vi "Table_ResizeListbox.vi"(7 "VI in":refnum<vi>, 8 "error in (no error)":errorcluster, 10 "Listbox Ref":refnum<vi>, 11 "State Information":T1) -> (0 "error out":errorcluster, 2 "Listbox Ref Out":refnum<vi>, 3 "State Information Out":T1)   [LabVIEW 2012, in "TableSupportLib.lvlib"]
uses:
  TableSupportLib.lvlib
  Table_StateInformation.ctl
  Table_ChannelInfoCluster.ctl
  Table_SortArraySettings.ctl
  Table_ListboxSettings.ctl
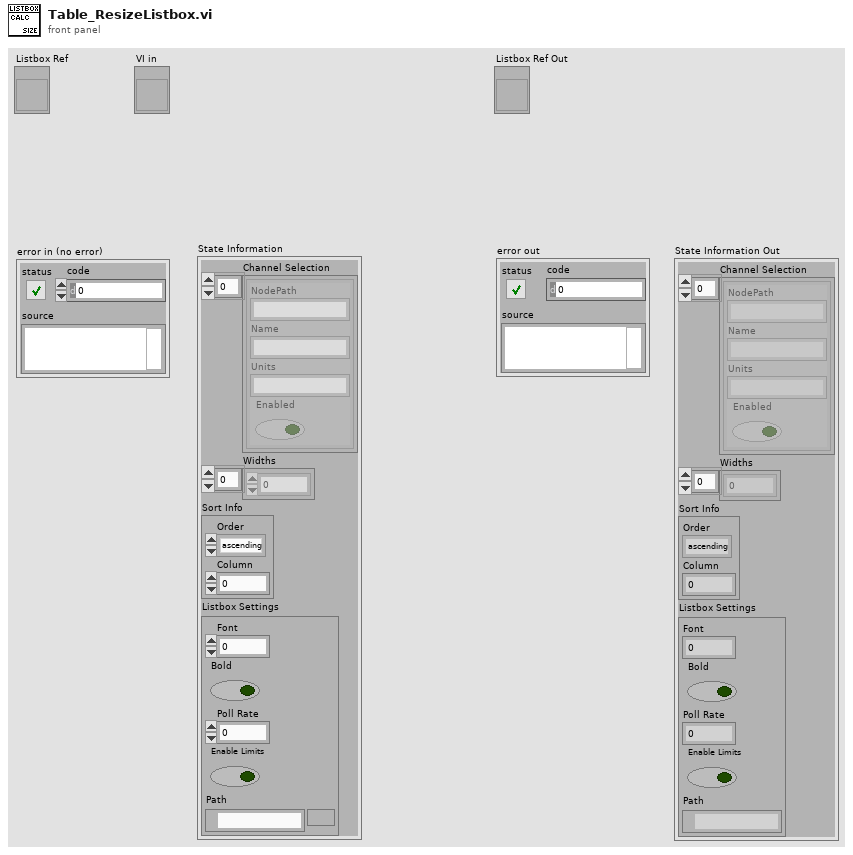
[diagram p1: front panel]
types:
  T1 = typedef "TableSupportLib.lvlib/Table_StateInformation.ctl" = cluster{"Channel Selection":T2[], "Widths":dbl[], "Sort Info":T3, "Listbox Settings":T4}
  T2 = typedef "TableSupportLib.lvlib/Table_ChannelInfoCluster.ctl" = cluster{"NodePath":string, "Name":string, "Units":string, "Enabled":bool}
  T3 = typedef "TableSupportLib.lvlib/Table_SortArraySettings.ctl" = cluster{"Order":enum16{"ascending", "descending"}, "Column":i32}
  T4 = typedef "TableSupportLib.lvlib/Table_ListboxSettings.ctl" = cluster{"Font":u32, "Bold":bool, "Poll Rate":u32, "Enable Limits":bool, "Path":path}
  T5 = typedef "LVBoundsTypeDef.ctl" = cluster{"Width":u32, "Height":u32}
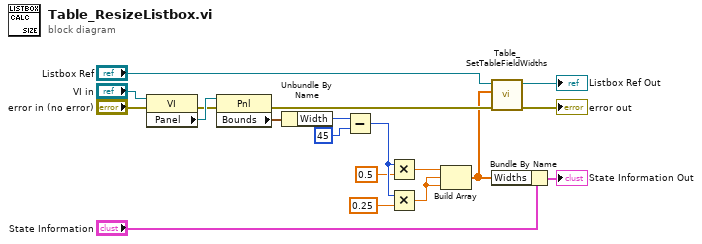
[diagram p0: block diagram]
diagram:
  n1 = property class="VI"(reference="VI in", error in="error in (no error)") -> (error out=w9:errorcluster, "Panel"=w19:refnum<vi>)  [unwired: 1 out]
  n2 = property class="Pnl"(reference=w19, error in=w9) -> (error out=w8:errorcluster, "Bounds"=w17:T5)  [unwired: 1 out]
  n3 = Unbundle By Name(w17) -> ("Width"=w16:u32)
  n4 = Subtract(x=w16, y=u32 45) -> (x-y=w14:u32)
  n5 = Multiply(x=w14, y=0.5) -> (x*y=w10:dbl)
  n6 = Multiply(x=w14, y=0.25) -> (x*y=w11:dbl)
  n7 = Build Array(w10, w11, w11) -> (w2:dbl[])
  n8 = call "Table_SetTableFieldWidths.vi"("error in (no error)"=w8, "Widths"=w2, "Listbox Ref"="Listbox Ref") -> ("error out"=→"error out":errorcluster, "Listbox Ref Out"=→"Listbox Ref Out":refnum<vi>)  [unwired: 7 in]
  n9 = Bundle By Name(cluster="State Information", "Widths"=w2) -> (→"State Information Out":T1)
